vi "数据发送组合-20200825 (子VI).vi"(10 "枚举":T2(ring), 11 "插值后的数组元素":T1) -> (3 "字符串":string)   [LabVIEW 2016, in "数据传输系统.lvlib"]
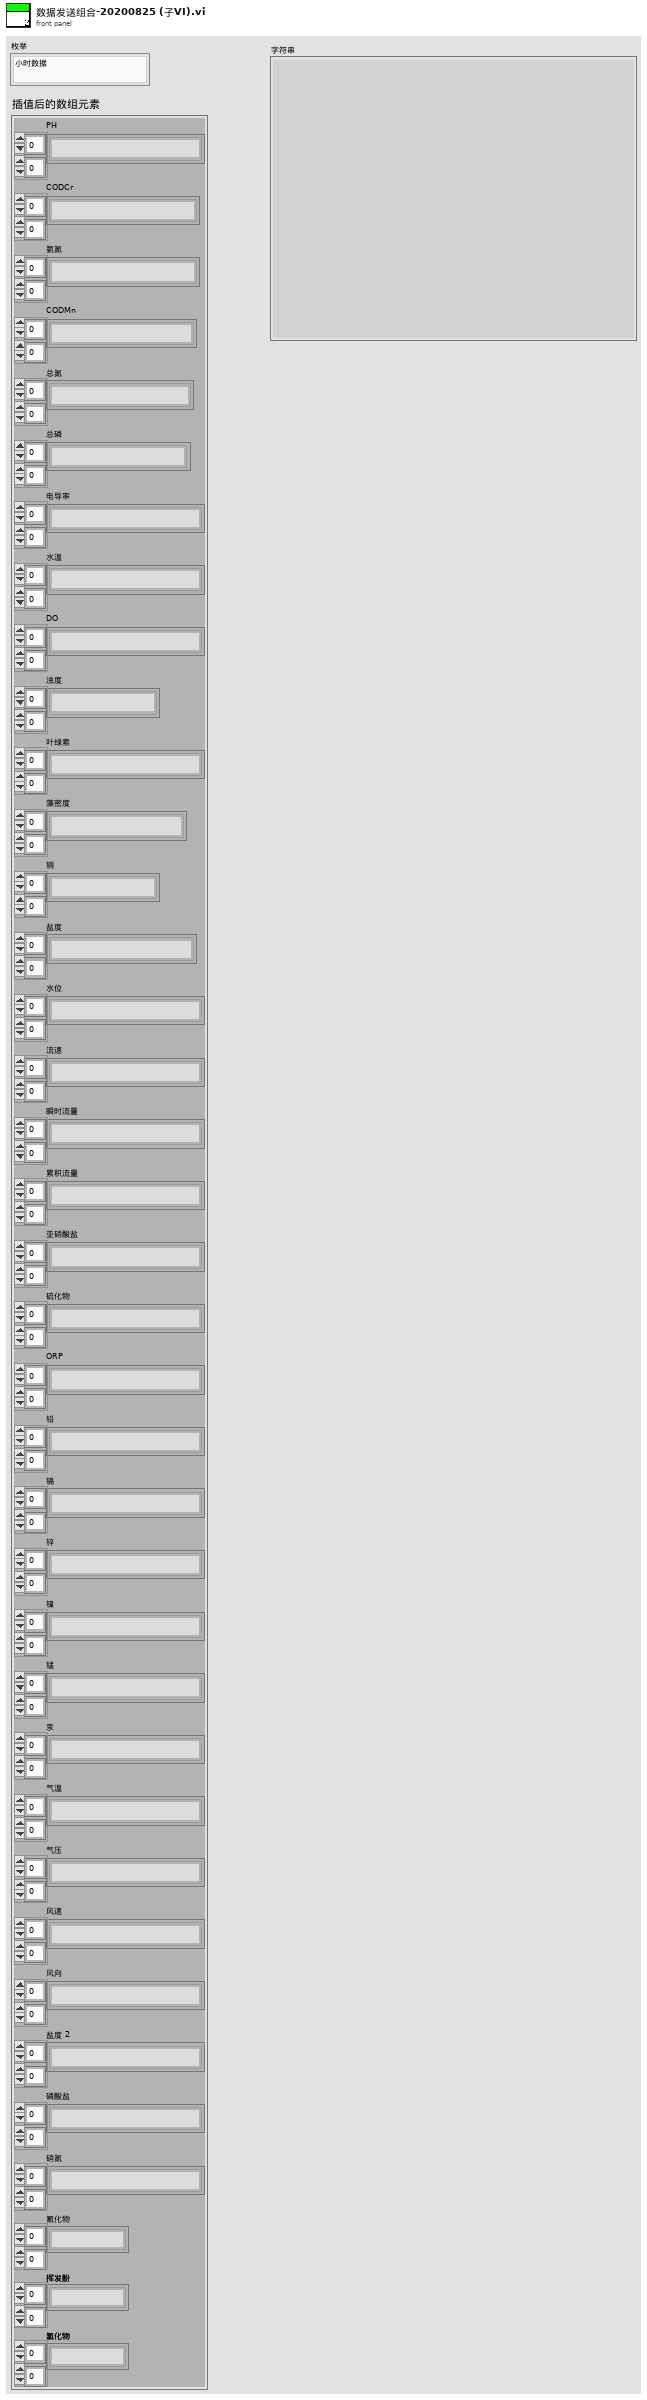
[diagram p1: front panel]
types:
  T1 = cluster{"PH":string[][], "CODCr":string[][], "氨氮":string[][], "CODMn":string[][], "总氮":string[][], "总磷":string[][], "电导率":string[][], "水温":string[][], "DO":string[][], "浊度":string[][], "叶绿素":string[][], "藻密度":string[][], "铜":string[][], "盐度":string[][], "水位":string[][], "流速":string[][], "瞬时流量":string[][], "累积流量":string[][], "亚硝酸盐":string[][], "硫化物":string[][], "ORP":string[][], "铅":string[][], "镉":string[][], "锌":string[][], "镍":string[][], "锰":string[][], "汞":string[][], "气温":string[][], "气压":string[][], "风速":string[][], "风向":string[][], "盐度 2":string[][], "磷酸盐":string[][], "硝氮":string[][], "氟化物":string[][], "挥发酚":string[][], "氯化物":string[][]}
  T2 = enum16{"小时数据", "实时数据", "平行样测试", "集成干预测试", "加标回收测试", "核查数据", "空白零点跨度数据", "提取小时数据", "提取实时数据", "操作日志", "仪器参数", "3090仪器参数", "提取仪器参数", "报警信息"}
  T3 = cluster{"CODMn":dbl, "CODCr":dbl, "DO":dbl, "铜":dbl, "PH":dbl, "氨氮":dbl, "比电导率":dbl, "水温":dbl, "COD":dbl, "浊度":dbl, "总氮":dbl, "总磷":dbl, "叶绿素a":dbl, "藻密度":dbl, "水位":dbl, "流速":dbl, "瞬时流量":dbl, "累积流量":dbl, "亚硝酸盐":dbl, "硫化物":dbl, "ORP":dbl, "铅":dbl, "镉":dbl, "锌":dbl, "镍":dbl, "锰":dbl, "汞":dbl, "气温":dbl, "气压":dbl, "风速":dbl, "风向":dbl, "盐度":dbl, "磷酸盐":dbl, "硝氮":dbl, "氟化物":dbl, "挥发酚":dbl, "氯化物":dbl}
  T4 = cluster{"CODMn":string, "CODCr":string, "DO":string, "铜":string, "PH":string, "氨氮":string, "比电导率":string, "水温":string, "COD":string, "浊度":string, "总氮":string, "总磷":string, "叶绿素a":string, "藻密度":string, "水位":string, "流速":string, "瞬时流量":string, "累积流量":string, "亚硝酸盐":string, "硫化物":string, "ORP":string, "铅":string, "镉":string, "锌":string, "镍":string, "锰":string, "汞":string, "气温":string, "气压":string, "风速":string, "风向":string, "盐度":string, "磷酸盐":string, "硝氮":string, "氟化物":string, "挥发酚":string, "氯化物":string}
  T5 = typedef "数据传输系统.lvlib/应用环境.ctl" = enum16{"STD", "GB212", "婉仪平台"}
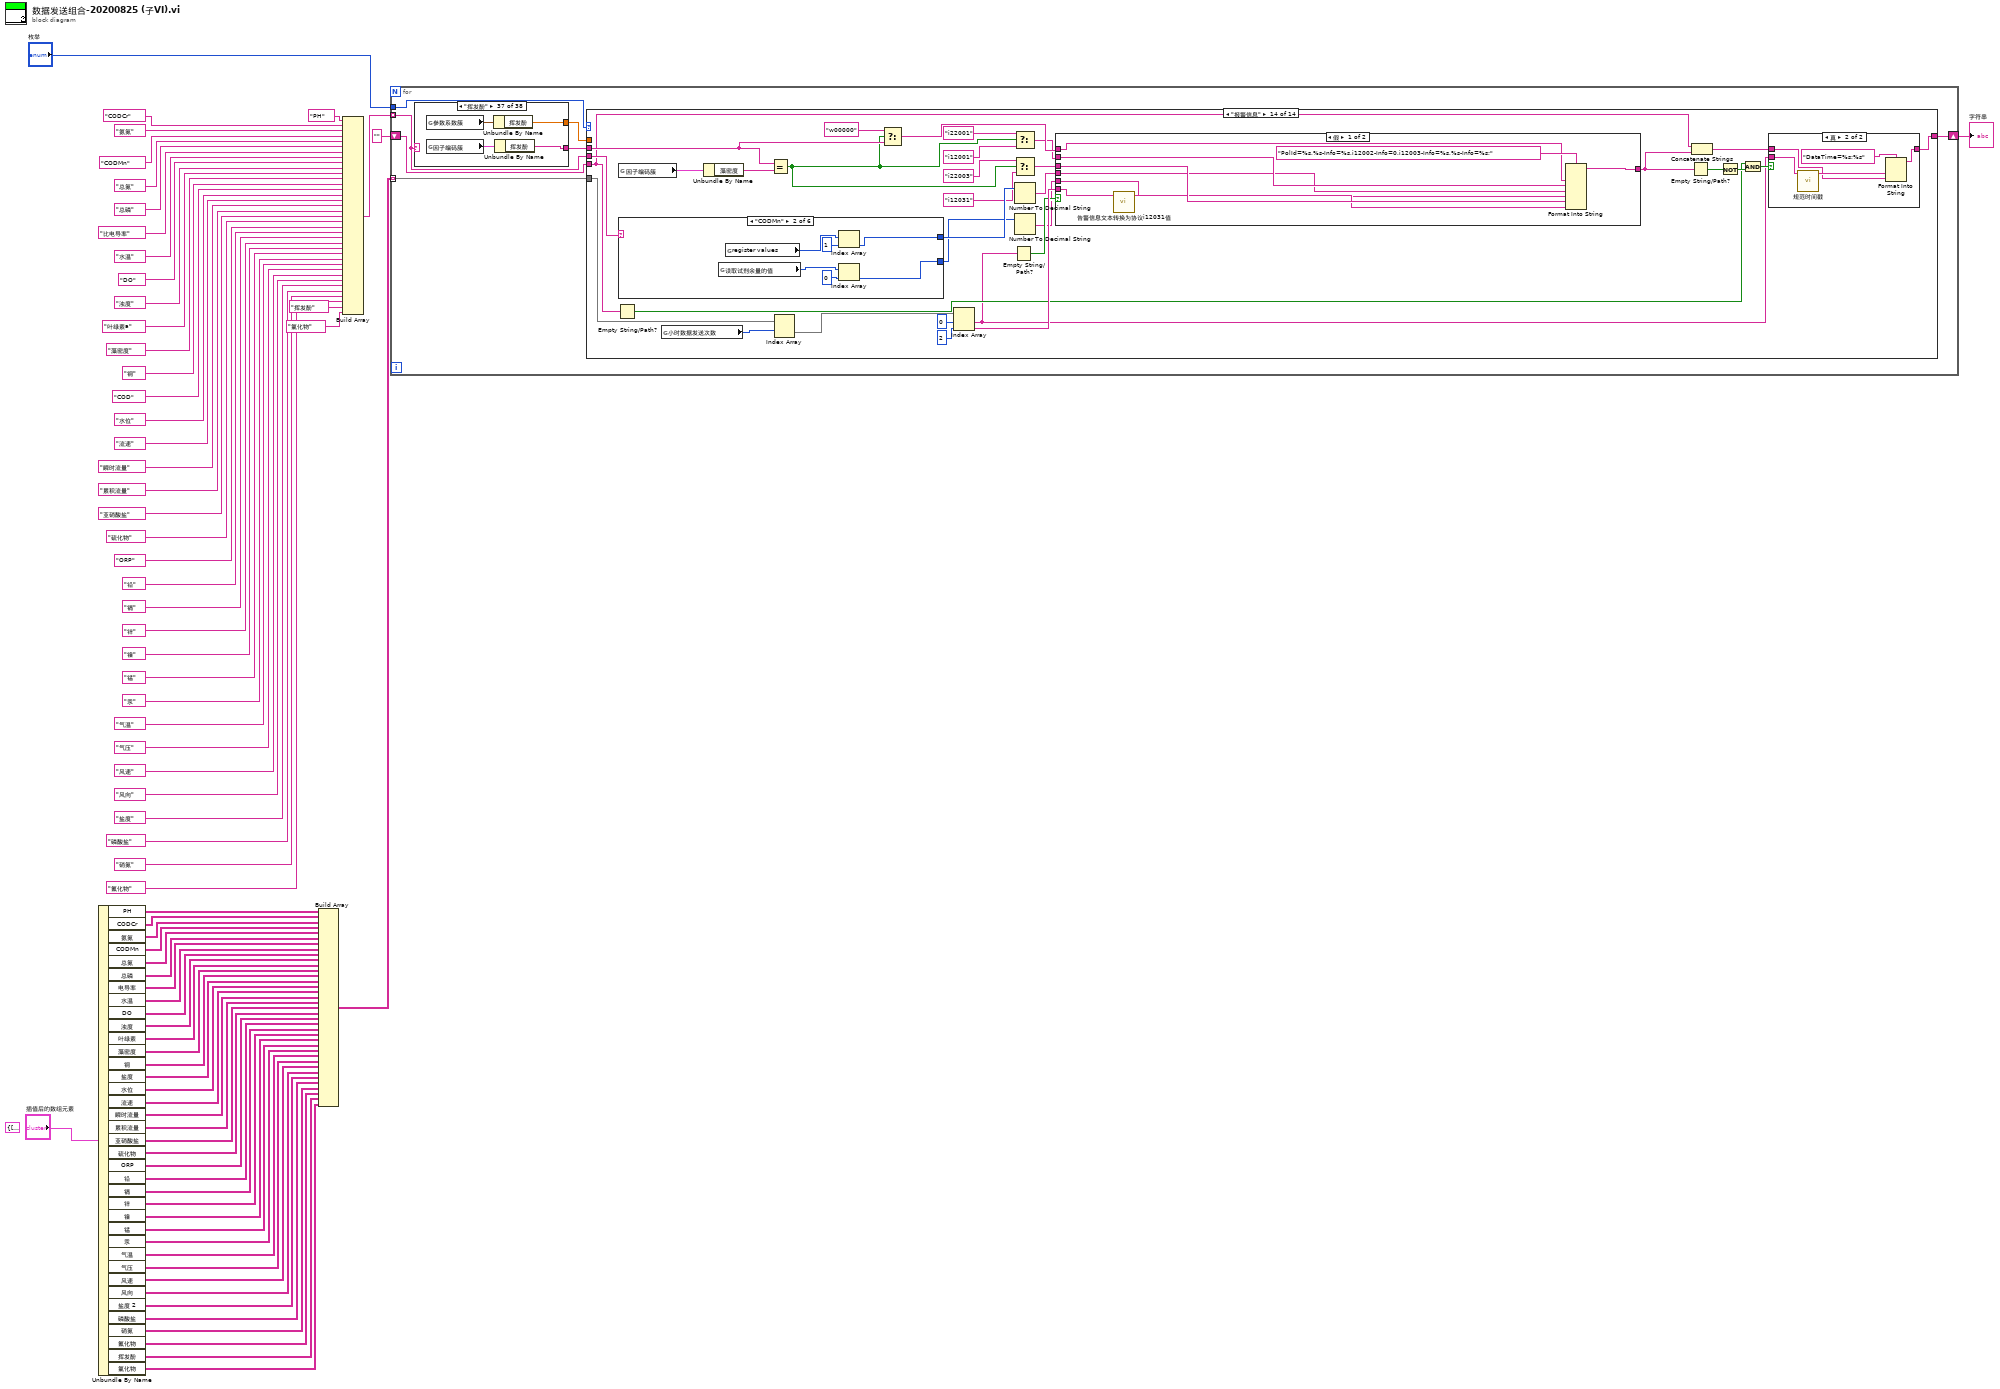
[diagram p0: block diagram]
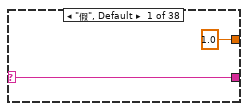
[diagram p2: hidden frame]
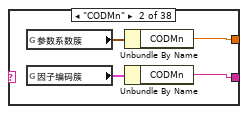
[diagram p3: hidden frame]
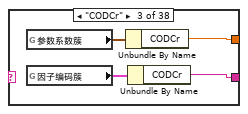
[diagram p4: hidden frame]
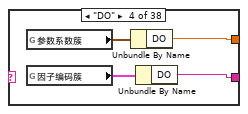
[diagram p5: hidden frame]
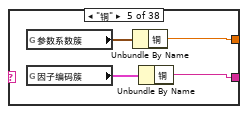
[diagram p6: hidden frame]
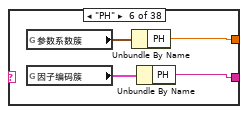
[diagram p7: hidden frame]
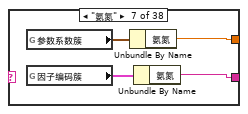
[diagram p8: hidden frame]
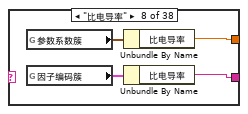
[diagram p9: hidden frame]
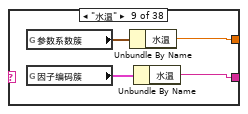
[diagram p10: hidden frame]
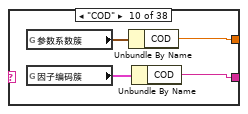
[diagram p11: hidden frame]
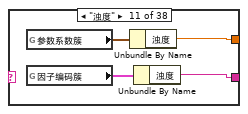
[diagram p12: hidden frame]
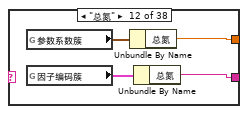
[diagram p13: hidden frame]
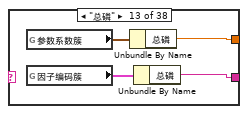
[diagram p14: hidden frame]
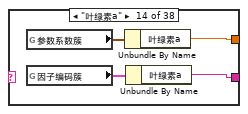
[diagram p15: hidden frame]
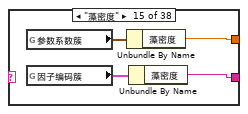
[diagram p16: hidden frame]
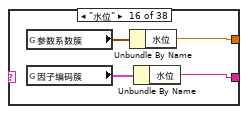
[diagram p17: hidden frame]
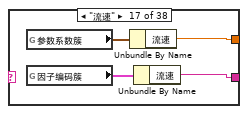
[diagram p18: hidden frame]
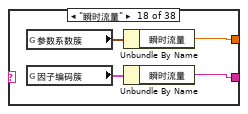
[diagram p19: hidden frame]
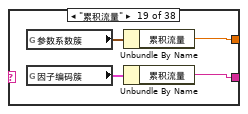
[diagram p20: hidden frame]
diagram:
  (unwired) T1 {"PH"=[], "CODCr"=[], "氨氮"=[], "CODMn"=[], "总氮"=[], "总磷"=[], "电导率"=[], "水温"=[], "DO"=[], "浊度"=[], "叶绿素"=[], "藻密度"=[], "铜"=[], "盐度"=[], "水位"=[], "流速"=[], "瞬时流量"=[], "累积流量"=[], "亚硝酸盐"=[], "硫化物"=[], "ORP"=[], "铅"=[], "镉"=[], "锌"=[], "镍"=[], "锰"=[], "汞"=[], "气温"=[], "气压"=[], "风速"=[], "风向"=[], "盐度 2"=[], "磷酸盐"=[], "硝氮"=[], "氟化物"=[], "挥发酚"=[], "氯化物"=[]} ("插值后的数组元素")
  n1 = Unbundle By Name("插值后的数组元素") -> ("PH"=w80:string[][], "CODCr"=w79:string[][], "氨氮"=w78:string[][], "CODMn"=w77:string[][], "总氮"=w76:string[][], "总磷"=w75:string[][], "电导率"=w74:string[][], "水温"=w73:string[][], "DO"=w72:string[][], "浊度"=w71:string[][], "叶绿素"=w70:string[][], "藻密度"=w69:string[][], "铜"=w68:string[][], "盐度"=w67:string[][], "水位"=w66:string[][], "流速"=w65:string[][], "瞬时流量"=w64:string[][], "累积流量"=w63:string[][], "亚硝酸盐"=w62:string[][], "硫化物"=w61:string[][], "ORP"=w60:string[][], "铅"=w59:string[][], "镉"=w58:string[][], "锌"=w57:string[][], "镍"=w56:string[][], "锰"=w55:string[][], "汞"=w54:string[][], "气温"=w18:string[][], "气压"=w19:string[][], "风速"=w20:string[][], "风向"=w21:string[][], "盐度 2"=w12:string[][], "磷酸盐"=w11:string[][], "硝氮"=w10:string[][], "氟化物"=w6:string[][], "挥发酚"=w4:string[][], "氯化物"=w3:string[][])
  n2 = Build Array(w80, w79, w78, w77, w76, w75, w74, w73, w72, w71, w70, w69, w68, w67, w66, w65, w64, w63, w62, w61, w60, w59, w58, w57, w56, w55, w54, w18, w19, w20, w21, w12, w11, w10, w6, w4, w3) -> (w53:string[][][])
  n3 = Build Array("PH" ("污染物编码"), "CODCr" ("污染物编码"), "氨氮" ("污染物编码"), "CODMn" ("污染物编码"), "总氮" ("污染物编码"), "总磷" ("污染物编码"), "比电导率" ("污染物编码"), "水温" ("污染物编码"), "DO" ("污染物编码"), "浊度" ("污染物编码"), "叶绿素a" ("污染物编码"), "藻密度" ("污染物编码"), "铜" ("污染物编码"), "COD" ("污染物编码"), "水位" ("污染物编码"), "流速" ("污染物编码"), "瞬时流量" ("污染物编码"), "累积流量" ("污染物编码"), "亚硝酸盐" ("污染物编码"), "硫化物" ("污染物编码"), "ORP" ("污染物编码"), "铅" ("污染物编码"), "镉" ("污染物编码"), "锌" ("污染物编码"), "镍" ("污染物编码"), "锰" ("污染物编码"), "汞" ("污染物编码"), "气温" ("污染物编码"), "气压" ("污染物编码"), "风速" ("污染物编码"), "风向" ("污染物编码"), "盐度" ("污染物编码"), "磷酸盐" ("污染物编码"), "硝氮" ("污染物编码"), "氟化物" ("污染物编码"), "挥发酚" ("污染物编码"), "氯化物" ("污染物编码")) -> (w25:string[])
  n4 = for {
    tunnel: w53 -> [w87] mode=indexing
    tunnel: w25 -> [w82] mode=indexing
    shift-right: [w86] -> w23
    shift-left: "" -> [w85]
    tunnel: "枚举" -> [w84]
    n5 = case shown="\"挥发酚\"" w82 {
      selector: w82 -> [w89 _ _ _ _ _ _ _ _ _ _ _ _ _ _ _ _ _ _ _ _ _ _ _ _ _ _ _ _ _ _ _ _ _ _ _ _ _]
      tunnel: [w89 w92 w96 w100 w104 w108 w112 w116 w120 w124 w128 w132 w136 w140 w144 w148 w152 w156 w160 w164 w168 w172 w176 w180 w184 w188 w192 w196 w200 w204 w208 w212 w216 w220 w224 w228 w232 w236] -> w83
      tunnel: [1.0 ("风向") w90 w94 w98 w102 w106 w110 w114 w118 w122 w126 w130 w134 w138 w142 w146 w150 w154 w158 w162 w166 w170 w174 w178 w182 w186 w190 w194 w198 w202 w206 w210 w214 w218 w222 w226 w230 w234] -> w81
      frame "假", Default {
      }
      frame "CODMn" {
        n6 = global read "断电保存全局.vi" "参数系数簇"() -> (w91:T3)
        n7 = global read "断电保存全局.vi" "因子编码簇"() -> (w93:T4)
        n8 = Unbundle By Name(w91) -> ("CODMn"=w90:dbl)
        n9 = Unbundle By Name(w93) -> ("CODMn"=w92:string)
      }
      frame "CODCr" {
        n10 = global read "断电保存全局.vi" "参数系数簇"() -> (w95:T3)
        n11 = global read "断电保存全局.vi" "因子编码簇"() -> (w97:T4)
        n12 = Unbundle By Name(w95) -> ("CODCr"=w94:dbl)
        n13 = Unbundle By Name(w97) -> ("CODCr"=w96:string)
      }
      frame "DO" {
        n14 = global read "断电保存全局.vi" "参数系数簇"() -> (w99:T3)
        n15 = global read "断电保存全局.vi" "因子编码簇"() -> (w101:T4)
        n16 = Unbundle By Name(w99) -> ("DO"=w98:dbl)
        n17 = Unbundle By Name(w101) -> ("DO"=w100:string)
      }
      frame "铜" {
        n18 = global read "断电保存全局.vi" "参数系数簇"() -> (w103:T3)
        n19 = global read "断电保存全局.vi" "因子编码簇"() -> (w105:T4)
        n20 = Unbundle By Name(w103) -> ("铜"=w102:dbl)
        n21 = Unbundle By Name(w105) -> ("铜"=w104:string)
      }
      frame "PH" {
        n22 = global read "断电保存全局.vi" "参数系数簇"() -> (w107:T3)
        n23 = global read "断电保存全局.vi" "因子编码簇"() -> (w109:T4)
        n24 = Unbundle By Name(w107) -> ("PH"=w106:dbl)
        n25 = Unbundle By Name(w109) -> ("PH"=w108:string)
      }
      frame "氨氮" {
        n26 = global read "断电保存全局.vi" "参数系数簇"() -> (w111:T3)
        n27 = global read "断电保存全局.vi" "因子编码簇"() -> (w113:T4)
        n28 = Unbundle By Name(w111) -> ("氨氮"=w110:dbl)
        n29 = Unbundle By Name(w113) -> ("氨氮"=w112:string)
      }
      frame "比电导率" {
        n30 = global read "断电保存全局.vi" "参数系数簇"() -> (w115:T3)
        n31 = global read "断电保存全局.vi" "因子编码簇"() -> (w117:T4)
        n32 = Unbundle By Name(w115) -> ("比电导率"=w114:dbl)
        n33 = Unbundle By Name(w117) -> ("比电导率"=w116:string)
      }
      frame "水温" {
        n34 = global read "断电保存全局.vi" "参数系数簇"() -> (w119:T3)
        n35 = global read "断电保存全局.vi" "因子编码簇"() -> (w121:T4)
        n36 = Unbundle By Name(w119) -> ("水温"=w118:dbl)
        n37 = Unbundle By Name(w121) -> ("水温"=w120:string)
      }
      frame "COD" {
        n38 = global read "断电保存全局.vi" "参数系数簇"() -> (w123:T3)
        n39 = global read "断电保存全局.vi" "因子编码簇"() -> (w125:T4)
        n40 = Unbundle By Name(w123) -> ("COD"=w122:dbl)
        n41 = Unbundle By Name(w125) -> ("COD"=w124:string)
      }
      frame "浊度" {
        n42 = global read "断电保存全局.vi" "参数系数簇"() -> (w127:T3)
        n43 = global read "断电保存全局.vi" "因子编码簇"() -> (w129:T4)
        n44 = Unbundle By Name(w127) -> ("浊度"=w126:dbl)
        n45 = Unbundle By Name(w129) -> ("浊度"=w128:string)
      }
      frame "总氮" {
        n46 = global read "断电保存全局.vi" "参数系数簇"() -> (w131:T3)
        n47 = global read "断电保存全局.vi" "因子编码簇"() -> (w133:T4)
        n48 = Unbundle By Name(w131) -> ("总氮"=w130:dbl)
        n49 = Unbundle By Name(w133) -> ("总氮"=w132:string)
      }
      frame "总磷" {
        n50 = global read "断电保存全局.vi" "参数系数簇"() -> (w135:T3)
        n51 = global read "断电保存全局.vi" "因子编码簇"() -> (w137:T4)
        n52 = Unbundle By Name(w135) -> ("总磷"=w134:dbl)
        n53 = Unbundle By Name(w137) -> ("总磷"=w136:string)
      }
      frame "叶绿素a" {
        n54 = global read "断电保存全局.vi" "参数系数簇"() -> (w139:T3)
        n55 = global read "断电保存全局.vi" "因子编码簇"() -> (w141:T4)
        n56 = Unbundle By Name(w139) -> ("叶绿素a"=w138:dbl)
        n57 = Unbundle By Name(w141) -> ("叶绿素a"=w140:string)
      }
      frame "藻密度" {
        n58 = global read "断电保存全局.vi" "参数系数簇"() -> (w143:T3)
        n59 = global read "断电保存全局.vi" "因子编码簇"() -> (w145:T4)
        n60 = Unbundle By Name(w143) -> ("藻密度"=w142:dbl)
        n61 = Unbundle By Name(w145) -> ("藻密度"=w144:string)
      }
      frame "水位" {
        n62 = global read "断电保存全局.vi" "参数系数簇"() -> (w147:T3)
        n63 = global read "断电保存全局.vi" "因子编码簇"() -> (w149:T4)
        n64 = Unbundle By Name(w147) -> ("水位"=w146:dbl)
        n65 = Unbundle By Name(w149) -> ("水位"=w148:string)
      }
      frame "流速" {
        n66 = global read "断电保存全局.vi" "参数系数簇"() -> (w151:T3)
        n67 = global read "断电保存全局.vi" "因子编码簇"() -> (w153:T4)
        n68 = Unbundle By Name(w151) -> ("流速"=w150:dbl)
        n69 = Unbundle By Name(w153) -> ("流速"=w152:string)
      }
      frame "瞬时流量" {
        n70 = global read "断电保存全局.vi" "参数系数簇"() -> (w155:T3)
        n71 = global read "断电保存全局.vi" "因子编码簇"() -> (w157:T4)
        n72 = Unbundle By Name(w155) -> ("瞬时流量"=w154:dbl)
        n73 = Unbundle By Name(w157) -> ("瞬时流量"=w156:string)
      }
      frame "累积流量" {
        n74 = global read "断电保存全局.vi" "参数系数簇"() -> (w159:T3)
        n75 = global read "断电保存全局.vi" "因子编码簇"() -> (w161:T4)
        n76 = Unbundle By Name(w159) -> ("累积流量"=w158:dbl)
        n77 = Unbundle By Name(w161) -> ("累积流量"=w160:string)
      }
      frame "亚硝酸盐" {
        n78 = global read "断电保存全局.vi" "参数系数簇"() -> (w163:T3)
        n79 = global read "断电保存全局.vi" "因子编码簇"() -> (w165:T4)
        n80 = Unbundle By Name(w163) -> ("亚硝酸盐"=w162:dbl)
        n81 = Unbundle By Name(w165) -> ("亚硝酸盐"=w164:string)
      }
      frame "硫化物" {
        n82 = global read "断电保存全局.vi" "参数系数簇"() -> (w167:T3)
        n83 = global read "断电保存全局.vi" "因子编码簇"() -> (w169:T4)
        n84 = Unbundle By Name(w167) -> ("硫化物"=w166:dbl)
        n85 = Unbundle By Name(w169) -> ("硫化物"=w168:string)
      }
      frame "ORP" {
        n86 = global read "断电保存全局.vi" "参数系数簇"() -> (w171:T3)
        n87 = global read "断电保存全局.vi" "因子编码簇"() -> (w173:T4)
        n88 = Unbundle By Name(w171) -> ("ORP"=w170:dbl)
        n89 = Unbundle By Name(w173) -> ("ORP"=w172:string)
      }
      frame "铅" {
        n90 = global read "断电保存全局.vi" "参数系数簇"() -> (w175:T3)
        n91 = global read "断电保存全局.vi" "因子编码簇"() -> (w177:T4)
        n92 = Unbundle By Name(w175) -> ("铅"=w174:dbl)
        n93 = Unbundle By Name(w177) -> ("铅"=w176:string)
      }
      frame "镉" {
        n94 = global read "断电保存全局.vi" "参数系数簇"() -> (w179:T3)
        n95 = global read "断电保存全局.vi" "因子编码簇"() -> (w181:T4)
        n96 = Unbundle By Name(w179) -> ("镉"=w178:dbl)
        n97 = Unbundle By Name(w181) -> ("镉"=w180:string)
      }
      frame "锌" {
        n98 = global read "断电保存全局.vi" "参数系数簇"() -> (w183:T3)
        n99 = global read "断电保存全局.vi" "因子编码簇"() -> (w185:T4)
        n100 = Unbundle By Name(w183) -> ("锌"=w182:dbl)
        n101 = Unbundle By Name(w185) -> ("锌"=w184:string)
      }
      frame "镍" {
        n102 = global read "断电保存全局.vi" "参数系数簇"() -> (w187:T3)
        n103 = global read "断电保存全局.vi" "因子编码簇"() -> (w189:T4)
        n104 = Unbundle By Name(w187) -> ("镍"=w186:dbl)
        n105 = Unbundle By Name(w189) -> ("镍"=w188:string)
      }
      frame "锰" {
        n106 = global read "断电保存全局.vi" "参数系数簇"() -> (w191:T3)
        n107 = global read "断电保存全局.vi" "因子编码簇"() -> (w193:T4)
        n108 = Unbundle By Name(w191) -> ("锰"=w190:dbl)
        n109 = Unbundle By Name(w193) -> ("锰"=w192:string)
      }
      frame "汞" {
        n110 = global read "断电保存全局.vi" "参数系数簇"() -> (w195:T3)
        n111 = global read "断电保存全局.vi" "因子编码簇"() -> (w197:T4)
        n112 = Unbundle By Name(w195) -> ("汞"=w194:dbl)
        n113 = Unbundle By Name(w197) -> ("汞"=w196:string)
      }
      frame "气温" {
        n114 = global read "断电保存全局.vi" "参数系数簇"() -> (w199:T3)
        n115 = global read "断电保存全局.vi" "因子编码簇"() -> (w201:T4)
        n116 = Unbundle By Name(w199) -> ("气温"=w198:dbl)
        n117 = Unbundle By Name(w201) -> ("气温"=w200:string)
      }
      frame "气压" {
        n118 = global read "断电保存全局.vi" "参数系数簇"() -> (w203:T3)
        n119 = global read "断电保存全局.vi" "因子编码簇"() -> (w205:T4)
        n120 = Unbundle By Name(w203) -> ("气压"=w202:dbl)
        n121 = Unbundle By Name(w205) -> ("气压"=w204:string)
      }
      frame "风速" {
        n122 = global read "断电保存全局.vi" "参数系数簇"() -> (w207:T3)
        n123 = global read "断电保存全局.vi" "因子编码簇"() -> (w209:T4)
        n124 = Unbundle By Name(w207) -> ("风速"=w206:dbl)
        n125 = Unbundle By Name(w209) -> ("风速"=w208:string)
      }
      frame "风向" {
        n126 = global read "断电保存全局.vi" "参数系数簇"() -> (w211:T3)
        n127 = global read "断电保存全局.vi" "因子编码簇"() -> (w213:T4)
        n128 = Unbundle By Name(w211) -> ("风向"=w210:dbl)
        n129 = Unbundle By Name(w213) -> ("风向"=w212:string)
      }
      frame "盐度" {
        n130 = global read "断电保存全局.vi" "参数系数簇"() -> (w215:T3)
        n131 = global read "断电保存全局.vi" "因子编码簇"() -> (w217:T4)
        n132 = Unbundle By Name(w215) -> ("盐度"=w214:dbl)
        n133 = Unbundle By Name(w217) -> ("盐度"=w216:string)
      }
      frame "磷酸盐" {
        n134 = global read "断电保存全局.vi" "参数系数簇"() -> (w219:T3)
        n135 = global read "断电保存全局.vi" "因子编码簇"() -> (w221:T4)
        n136 = Unbundle By Name(w219) -> ("磷酸盐"=w218:dbl)
        n137 = Unbundle By Name(w221) -> ("磷酸盐"=w220:string)
      }
      frame "硝氮" {
        n138 = global read "断电保存全局.vi" "参数系数簇"() -> (w223:T3)
        n139 = global read "断电保存全局.vi" "因子编码簇"() -> (w225:T4)
        n140 = Unbundle By Name(w223) -> ("硝氮"=w222:dbl)
        n141 = Unbundle By Name(w225) -> ("硝氮"=w224:string)
      }
      frame "氟化物" {
        n142 = global read "断电保存全局.vi" "参数系数簇"() -> (w227:T3)
        n143 = global read "断电保存全局.vi" "因子编码簇"() -> (w229:T4)
        n144 = Unbundle By Name(w227) -> ("氟化物"=w226:dbl)
        n145 = Unbundle By Name(w229) -> ("氟化物"=w228:string)
      }
      frame "挥发酚" {
        n146 = global read "断电保存全局.vi" "参数系数簇"() -> (w231:T3)
        n147 = global read "断电保存全局.vi" "因子编码簇"() -> (w233:T4)
        n148 = Unbundle By Name(w231) -> ("挥发酚"=w230:dbl)
        n149 = Unbundle By Name(w233) -> ("挥发酚"=w232:string)
      }
      frame "氯化物" {
        n150 = global read "断电保存全局.vi" "参数系数簇"() -> (w235:T3)
        n151 = global read "断电保存全局.vi" "因子编码簇"() -> (w237:T4)
        n152 = Unbundle By Name(w235) -> ("氯化物"=w234:dbl)
        n153 = Unbundle By Name(w237) -> ("氯化物"=w236:string)
      }
    }
    n154 = case shown="\"报警信息\"" w84 {
      tunnel: w87 -> [w252 w297 w328 w337 w392 w398 w410 w434 w456 w493 w511 w518 w528 w550]
      tunnel: w83 -> [w248 w290 w327 w338 w388 w397 w409 w428 w455 w481 w509 w516 w527 w553]
      tunnel: [w251 w294 w329 w335 w393 w394 w406 w425 w454 w488 w506 w515 w523 w539] -> w86
      tunnel: w85 -> [w250 w295 w331 w336 w389 w396 w407 w426 w457 w489 w507 w517 w524 w534]
      tunnel: w82 -> [w246 w289 _ w332 _ _ _ _ _ _ _ _ _ w548]
      tunnel: w81 -> [w243 w285 _ w333 _ _ _ w421 w450 _ _ _ _ _]
      frame "小时数据", Default {
        n155 = global read "全局 小时数据发送次数.vi" "小时数据发送次数"() -> (w255:i32)
        n156 = Index Array(array=w252, index (row)=w255) -> (element=w254:string[])  [unwired: 1 in]
        n157 = case shown="\"\", 默认" w246 {
          tunnel: w254 -> [w267 w270]
          tunnel: [w264 w268] -> w244
          tunnel: ["N" ("字符串") w269] -> w240
          frame "风速", "风向", "累积流量", "流速", "气温", "气压", "水位", "瞬时流量" {
            n158 = Index Array(array=w267, index=1 ("索引")) -> (element=w264:string)
          }
          frame "", Default {
            n159 = Index Array(array=w270, index #1=2 ("索引"), index #2=3 ("索引"), index #3=5 ("索引")) -> (element #1=w273:string, element #2=w272:string, element #3=w269:string)
            n160 = case shown="\"N\", 默认" w273 {
              tunnel: [w276 ""] -> w268
              tunnel: w272 -> [w276 _]
              frame "N", Default {
              }
              frame "M" {
              }
            }
          }
        }
        n161 = Empty String/Path?(string/path=w244) -> (empty?=w245:bool)
        n162 = case shown="假" w245 {
          tunnel: w244 -> [w261 w263]
          tunnel: w243 -> [w260 _]
          tunnel: [w258 w263] -> w242
          frame False {
            n163 = Fract/Exp String To Number(string=w261) -> (number=w262:dbl)  [unwired: 3 in, 1 out]
            n164 = Multiply(x=w262, y=w260) -> (x*y=w259:dbl)
            n165 = Number To Fractional String(number=w259) -> (F-format string=w258:string)  [unwired: 3 in]
          }
          frame True {
            # "空"
          }
        }
        n166 = global read "断电保存全局.vi" "地表水/污染源"() -> (w241:bool)
        n167 = call "数据编码整合输出.vi"("数据标识"=w240, "数据类型"="-Avg=", "污染物编码"=w248, "地表水/污染源"=w241, "数据值"=w242) -> ("编码输出"=w239:string)  [unwired: 6 in]
        n168 = case shown="\"pf\"" w240 {
          tunnel: w239 -> [w256 _]
          tunnel: [w256 ""] -> w238
          frame "假", Default {
          }
          frame "pf" {
            # "pf不传小时数据"
          }
        }
        n169 = global read "断电保存全局.vi" "数据发送协议"() -> (w249:enum16{"2005-212协议", "2017-212协议"})
        n170 = case shown="\"2017-212协议\"" w249 {
          tunnel: w246 -> [w280 _]
          tunnel: w238 -> [w278 w283]
          tunnel: [w279 w283] -> w247
          frame "2005-212协议", Default {
            n171 = case shown="\"风速\", \"风向\", \"累积流量\", \"流速\", \"气温\", \"气压\", \"水位\"" w280 {
              tunnel: [w281 ""] -> w279
              tunnel: w278 -> [w281 _]
              frame "假", Default {
              }
              frame "风速", "风向", "累积流量", "流速", "气温", "气压", "水位" {
              }
            }
          }
          frame "2017-212协议" {
          }
        }
        n172 = Concatenate Strings(w250, w247) -> (w251:string)
      }
      frame "实时数据" {
        n173 = global read "全局 小时数据发送次数.vi" "小时数据发送次数"() -> (w298:i32)
        n174 = Index Array(array=w297, index (row)=w298) -> (element=w299:string[])  [unwired: 1 in]
        n175 = case shown="\"\", 默认" w289 {
          tunnel: w299 -> [w308 w312 w318]
          tunnel: [w307 w311 w317] -> w287
          tunnel: ["N" ("字符串") "N" ("字符串") w315] -> w296
          frame "累积流量", "流速", "水位", "瞬时流量" {
            n176 = Index Array(array=w308, index=1 ("索引")) -> (element=w307:string)
          }
          frame "风速", "风向", "气温", "气压" {
            n177 = Index Array(array=w312, index=1 ("索引")) -> (element=w311:string)
          }
          frame "", Default {
            n178 = Index Array(array=w318, index #1=3 ("索引"), index #2=5 ("索引")) -> (element #1=w317:string, element #2=w315:string)
          }
        }
        n179 = Empty String/Path?(string/path=w287) -> (empty?=w288:bool)
        n180 = case shown="假" w288 {
          tunnel: w287 -> [w304 w306]
          tunnel: w285 -> [w303 _]
          tunnel: [w301 w306] -> w286
          frame False {
            n181 = Fract/Exp String To Number(string=w304) -> (number=w305:dbl)  [unwired: 3 in, 1 out]
            n182 = Multiply(x=w305, y=w303) -> (x*y=w302:dbl)
            n183 = Number To Fractional String(number=w302) -> (F-format string=w301:string)  [unwired: 3 in]
          }
          frame True {
            # "空"
          }
        }
        n184 = global read "断电保存全局.vi" "数据发送协议"() -> (w293:enum16{"2005-212协议", "2017-212协议"})
        n185 = call "数据编码整合输出.vi"("数据标识"=w296, "数据类型"="-Rtd=", "污染物编码"=w290, "地表水/污染源"=FALSE, "数据值"=w286) -> ("编码输出"=w292:string)  [unwired: 6 in]
        n186 = case shown="\"2017-212协议\"" w293 {
          tunnel: w289 -> [w322 _]
          tunnel: w292 -> [w320 w325]
          tunnel: [w321 w325] -> w291
          frame "2005-212协议", Default {
            n187 = case shown="\"假\", 默认" w322 {
              tunnel: [w323 ""] -> w321
              tunnel: w320 -> [w323 _]
              frame "假", Default {
              }
              frame "风速", "风向", "累积流量", "流速", "气温", "气压", "水位" {
              }
            }
          }
          frame "2017-212协议" {
          }
        }
        n188 = Concatenate Strings(w295, w291) -> (w294:string)
      }
      frame "平行样测试" {
        n189 = global read "全局 小时数据发送次数.vi" "小时数据发送次数"() -> (w326:i32)
        n190 = call "平行样集成干预数据组合(子VI).vi"("污染物编码"=w327, "数据输入"=w328, "小时数据发送次数"=w326) -> ("输出组合"=w330:string)  [unwired: 8 in]
        n191 = Concatenate Strings(w331, w330) -> (w329:string)
      }
      frame "集成干预测试" {
        n192 = global read "断电保存全局.vi" "应用环境"() -> (w334:T5)
        n193 = case shown="\"GB212\", 默认" w334 {
          tunnel: w338 -> [w342 w348]
          tunnel: w337 -> [w341 w349]
          tunnel: w336 -> [w340 w350]
          tunnel: [w339 w345] -> w335
          tunnel: w333 -> [_ w347]
          tunnel: w332 -> [_ w346]
          frame "STD" {
            n194 = global read "全局 小时数据发送次数.vi" "小时数据发送次数"() -> (w343:i32)
            n195 = call "平行样集成干预数据组合(子VI).vi"("污染物编码"=w342, "数据输入"=w341, "小时数据发送次数"=w343) -> ("输出组合"=w344:string)  [unwired: 8 in]
            n196 = Concatenate Strings(w340, w344) -> (w339:string)
          }
          frame "GB212", Default {
            n197 = global read "全局 小时数据发送次数.vi" "小时数据发送次数"() -> (w361:i32)
            n198 = Index Array(array=w349, index (row)=w361) -> (element=w360:string[])  [unwired: 1 in]
            n199 = case shown="\"\", 默认" w346 {
              tunnel: w360 -> [w371 w374]
              tunnel: [w368 w373] -> w353
              tunnel: ["N" ("字符串") w372] -> w358
              frame "风速", "风向", "累积流量", "流速", "气温", "气压", "水位", "瞬时流量" {
                n200 = Index Array(array=w371, index=1 ("索引")) -> (element=w368:string)
              }
              frame "", Default {
                n201 = Index Array(array=w374, index #1=2 ("索引"), index #2=3 ("索引"), index #3=5 ("索引")) -> (element #1=w377:string, element #2=w376:string, element #3=w372:string)
                n202 = case shown="\"N\", 默认" w377 {
                  tunnel: [w380 ""] -> w373
                  tunnel: w376 -> [w380 _]
                  frame "N", Default {
                  }
                  frame "M" {
                  }
                }
              }
            }
            n203 = Empty String/Path?(string/path=w353) -> (empty?=w354:bool)
            n204 = case shown="假" w354 {
              tunnel: w353 -> [w365 w367]
              tunnel: w347 -> [w364 _]
              tunnel: [w362 w367] -> w352
              frame False {
                n205 = Fract/Exp String To Number(string=w365) -> (number=w366:dbl)  [unwired: 3 in, 1 out]
                n206 = Multiply(x=w366, y=w364) -> (x*y=w363:dbl)
                n207 = Number To Fractional String(number=w363) -> (F-format string=w362:string)  [unwired: 3 in]
              }
              frame True {
                # "空"
              }
            }
            n208 = global read "断电保存全局.vi" "地表水/污染源"() -> (w351:bool)
            n209 = global read "断电保存全局.vi" "数据发送协议"() -> (w357:enum16{"2005-212协议", "2017-212协议"})
            n210 = call "数据编码整合输出.vi"("数据标识"=w358, "数据类型"="-Avg=", "污染物编码"=w348, "地表水/污染源"=w351, "数据值"=w352) -> ("编码输出"=w356:string)  [unwired: 6 in]
            n211 = case shown="\"2017-212协议\"" w357 {
              tunnel: w346 -> [w384 _]
              tunnel: w356 -> [w382 w387]
              tunnel: [w383 w387] -> w355
              frame "2005-212协议", Default {
                n212 = case shown="\"假\", 默认" w384 {
                  tunnel: [w385 ""] -> w383
                  tunnel: w382 -> [w385 _]
                  frame "假", Default {
                  }
                  frame "风速", "风向", "累积流量", "流速", "气温", "气压", "水位" {
                  }
                }
              }
              frame "2017-212协议" {
              }
            }
            n213 = Concatenate Strings(w350, w355) -> (w345:string)
          }
        }
      }
      frame "加标回收测试" {
        n214 = global read "全局 小时数据发送次数.vi" "小时数据发送次数"() -> (w391:i32)
        n215 = call "加标回收数据组合 (子VI).vi"("小时数据发送次数"=w391, "数据"=w392, "污染物编码"=w388) -> ("组合输出"=w390:string)  [unwired: 7 in, 1 out]
        n216 = Concatenate Strings(w389, w390) -> (w393:string)
      }
      frame "核查数据" {
        n217 = global read "全局 小时数据发送次数.vi" "小时数据发送次数"() -> (w399:i32)
        n218 = call "标样核查数据组合(子VI).vi"("小时数据发送次数"=w399, "数据输入"=w398, "污染物编码"=w397) -> ("输出组合"=w395:string)  [unwired: 8 in]
        n219 = Concatenate Strings(w396, w395) -> (w394:string)
      }
      frame "空白零点跨度数据" {
        n220 = global read "全局 小时数据发送次数.vi" "小时数据发送次数"() -> (w412:i32)
        n221 = Index Array(array=w410, index (row)=w412) -> (element=w416:string[])  [unwired: 1 in]
        n222 = Index Array(array=w416, index #1=0 ("索引"), index #2=3 ("索引"), index #3=6 ("索引"), index #4=7 ("索引"), index #5=5 ("索引")) -> (element #2=w411:string, element #3=w413:string, element #4=w402:string, element #5=w400:string)  [unwired: 1 out]
        n223 = Empty String/Path?(string/path=w402) -> (empty?=w404:bool)
        n224 = case shown="假" w404 {
          tunnel: [w418 "0" ("span value")] -> w403
          tunnel: w402 -> [w418 _]
          frame False {
          }
          frame True {
          }
        }
        n225 = call "零点跨度数据组合 (子VI).vi"("数据标识"=w400, "span value"=w403, "standard value"=w413, "check value"=w411, "污染物编码"=w409) -> ("组合输出"=w408:string)  [unwired: 6 in]
        n226 = Concatenate Strings(w407, w408) -> (w406:string)
      }
      frame "提取小时数据" {
        n227 = global read "全局 小时数据发送次数.vi" "小时数据发送次数"() -> (w435:i32)
        n228 = Index Array(array=w434, index (row)=w435) -> (element=w433:string[])  [unwired: 1 in]
        n229 = Index Array(array=w433, index #2=1 ("索引")) -> (element #2=w422:string)  [unwired: 1 in, 1 out]
        n230 = Empty String/Path?(string/path=w422) -> (empty?=w424:bool)
        n231 = case shown="假" w424 {
          tunnel: w422 -> [w440 w442]
          tunnel: w421 -> [w439 _]
          tunnel: [w437 w442] -> w423
          frame False {
            n232 = Fract/Exp String To Number(string=w440) -> (number=w441:dbl)  [unwired: 3 in, 1 out]
            n233 = Multiply(x=w441, y=w439) -> (x*y=w438:dbl)
            n234 = Number To Fractional String(number=w438) -> (F-format string=w437:string)  [unwired: 3 in]
          }
          frame True {
            # "空"
          }
        }
        n235 = global read "断电保存全局.vi" "地表水/污染源"() -> (w420:bool)
        n236 = global read "断电保存全局.vi" "数据发送协议"() -> (w430:enum16{"2005-212协议", "2017-212协议"})
        n237 = call "数据编码整合输出.vi"("数据标识"="N", "数据类型"="-Avg=", "污染物编码"=w428, "地表水/污染源"=w420, "数据值"=w423) -> ("编码输出"=w427:string)  [unwired: 6 in]
        n238 = case shown="\"2005-212协议\", 默认" w430 {
          tunnel: w428 -> [w445 _]
          tunnel: w427 -> [w443 w448]
          tunnel: [w444 w448] -> w429
          frame "2005-212协议", Default {
            n239 = case shown="\"假\", 默认" w445 {
              tunnel: [w446 ""] -> w444
              tunnel: w443 -> [w446 _]
              frame "假", Default {
              }
              frame "累积流量", "流速", "水位" {
              }
            }
          }
          frame "2017-212协议" {
          }
        }
        n240 = Concatenate Strings(w426, w429) -> (w425:string)
      }
      frame "提取实时数据" {
        n241 = global read "全局 小时数据发送次数.vi" "小时数据发送次数"() -> (w463:i32)
        n242 = Index Array(array=w456, index (row)=w463) -> (element=w464:string[])  [unwired: 1 in]
        n243 = Index Array(array=w464, index #1=3 ("索引"), index #2=5 ("索引")) -> (element #1=w451:string, element #2=w461:string)
        n244 = Empty String/Path?(string/path=w451) -> (empty?=w453:bool)
        n245 = case shown="假" w453 {
          tunnel: w451 -> [w470 w472]
          tunnel: w450 -> [w469 _]
          tunnel: [w467 w472] -> w452
          frame False {
            n246 = Fract/Exp String To Number(string=w470) -> (number=w471:dbl)  [unwired: 3 in, 1 out]
            n247 = Multiply(x=w471, y=w469) -> (x*y=w468:dbl)
            n248 = Number To Fractional String(number=w468) -> (F-format string=w467:string)  [unwired: 3 in]
          }
          frame True {
            # "空"
          }
        }
        n249 = global read "断电保存全局.vi" "地表水/污染源"() -> (w449:bool)
        n250 = global read "断电保存全局.vi" "数据发送协议"() -> (w460:enum16{"2005-212协议", "2017-212协议"})
        n251 = call "数据编码整合输出.vi"("数据标识"=w461, "数据类型"="-Rtd=", "污染物编码"=w455, "地表水/污染源"=w449, "数据值"=w452) -> ("编码输出"=w459:string)  [unwired: 6 in]
        n252 = case shown="\"2017-212协议\"" w460 {
          tunnel: w455 -> [w475 _]
          tunnel: w459 -> [w473 w478]
          tunnel: [w474 w478] -> w458
          frame "2005-212协议", Default {
            n253 = case shown="\"累积流量\", \"流速\", \"水位\"" w475 {
              tunnel: [w476 ""] -> w474
              tunnel: w473 -> [w476 _]
              frame "假", Default {
              }
              frame "累积流量", "流速", "水位" {
              }
            }
          }
          frame "2017-212协议" {
          }
        }
        n254 = Concatenate Strings(w457, w458) -> (w454:string)
      }
      frame "操作日志" {
        n255 = global read "断电保存全局.vi" "因子编码簇"() -> (w484:T4)
        n256 = global read "全局 小时数据发送次数.vi" "小时数据发送次数"() -> (w497:i32)
        n257 = Unbundle By Name(w484) -> ("DO"=w483:string)
        n258 = Equal?(x=w481, y=w483) -> (x = y?=w479:bool)
        n259 = Index Array(array=w493, index (row)=w497) -> (element=w492:string[])  [unwired: 1 in]
        n260 = Index Array(array=w492, index #1=0 ("索引"), index #2=2 ("索引")) -> (element #2=w491:string)  [unwired: 1 out]
        n261 = Empty String/Path?(string/path=w491) -> (empty?=w496:bool)
        n262 = Select(t="w00000", s=w479, f=w481) -> (s? t:f=w480:string)
        n263 = Select(t="i21001", s=w479, f="i11001") -> (s? t:f=w485:string)
        n264 = case shown="假" w496 {
          tunnel: [w501 ""] -> w490
          tunnel: w491 -> [w499 _]
          tunnel: w480 -> [w500 _]
          tunnel: w485 -> [w498 _]
          frame False {
            n265 = Format Into String(format string="PolId=%s,%s-Info=//%s//;" ("格式字符串"), w500, w498, w499) -> (resulting string=w501:string)  [unwired: 2 in, 1 out]
          }
          frame True {
          }
        }
        n266 = Concatenate Strings(w489, w490) -> (w488:string)
      }
      frame "仪器参数" {
        n267 = global read "断电保存全局.vi" "应用环境"() -> (w505:T5)
        n268 = global read "全局 小时数据发送次数.vi" "小时数据发送次数"() -> (w512:i32)
        n269 = case shown="\"GB212\", 默认" w505 {
          tunnel: ["3090仪器参数" ("table") "仪器参数" ("table")] -> w504
          frame "STD" {
          }
          frame "GB212", Default {
          }
        }
        n270 = Index Array(array=w511, index (row)=w512) -> (element=w510:string[])  [unwired: 1 in]
        n271 = call "关键参数组合 (子VI).vi"("table"=w504, "因子编码"=w509, "data"=w510) -> ("字符串"=w508:string)  [unwired: 8 in]
        n272 = Concatenate Strings(w507, w508) -> (w506:string)
      }
      frame "3090仪器参数" {
        n273 = global read "全局 小时数据发送次数.vi" "小时数据发送次数"() -> (w522:i32)
        n274 = Index Array(array=w518, index (row)=w522) -> (element=w520:string[])  [unwired: 1 in]
        n275 = call "关键参数组合 (子VI).vi"("table"="3090仪器参数", "因子编码"=w516, "data"=w520) -> ("字符串"=w519:string)  [unwired: 8 in]
        n276 = Concatenate Strings(w517, w519) -> (w515:string)
      }
      frame "提取仪器参数" {
        n277 = global read "全局 小时数据发送次数.vi" "小时数据发送次数"() -> (w529:i32)
        n278 = Index Array(array=w528, index (row)=w529) -> (element=w526:string[])  [unwired: 1 in]
        n279 = call "提取仪器参数 (子VI).vi"("因子编码"=w527, "数据输入"=w526) -> ("字符串"=w525:string)  [unwired: 9 in]
        n280 = Concatenate Strings(w524, w525) -> (w523:string)
      }
      frame "报警信息" {
        n281 = Empty String/Path?(string/path=w534) -> (empty?=w533:bool)
        n282 = global read "断电保存全局.vi" "因子编码簇"() -> (w556:T4)
        n283 = case shown="\"CODMn\"" w548 {
          tunnel: [u16 0 ("register") w574 w580 w586 w592 w598] -> w546
          tunnel: [u16 0 ("register") w571 w577 w583 w589 w595] -> w531
          frame "假", Default {
          }
          frame "CODMn" {
            n284 = global read "全局1.vi" "读取试剂余量的值"() -> (w572:u16[])
            n285 = global read "全局1.vi" "register values"() -> (w576:u16[])
            n286 = Index Array(array=w576, index=1 ("索引")) -> (element=w574:u16)
            n287 = Index Array(array=w572, index=0 ("索引")) -> (element=w571:u16)
          }
          frame "氨氮" {
            n288 = global read "全局1.vi" "读取试剂余量的值"() -> (w578:u16[])
            n289 = global read "全局1.vi" "register values"() -> (w582:u16[])
            n290 = Index Array(array=w582, index=2 ("索引")) -> (element=w580:u16)
            n291 = Index Array(array=w578, index=1 ("索引")) -> (element=w577:u16)
          }
          frame "总磷" {
            n292 = global read "全局1.vi" "读取试剂余量的值"() -> (w584:u16[])
            n293 = global read "全局1.vi" "register values"() -> (w588:u16[])
            n294 = Index Array(array=w588, index=3 ("索引")) -> (element=w586:u16)
            n295 = Index Array(array=w584, index=2 ("索引")) -> (element=w583:u16)
          }
          frame "总氮" {
            n296 = global read "全局1.vi" "读取试剂余量的值"() -> (w590:u16[])
            n297 = global read "全局1.vi" "register values"() -> (w594:u16[])
            n298 = Index Array(array=w594, index=4 ("索引")) -> (element=w592:u16)
            n299 = Index Array(array=w590, index=3 ("索引")) -> (element=w589:u16)
          }
          frame "CODCr" {
            n300 = global read "全局1.vi" "读取试剂余量的值"() -> (w596:u16[])
            n301 = global read "全局1.vi" "register values"() -> (w600:u16[])
            n302 = Index Array(array=w600, index=5 ("索引")) -> (element=w598:u16)
            n303 = Index Array(array=w596, index=4 ("索引")) -> (element=w595:u16)
          }
        }
        n304 = global read "全局 小时数据发送次数.vi" "小时数据发送次数"() -> (w551:i32)
        n305 = Unbundle By Name(w556) -> ("藻密度"=w555:string)
        n306 = Equal?(x=w553, y=w555) -> (x = y?=w543:bool)
        n307 = Index Array(array=w550, index (row)=w551) -> (element=w549:string[])  [unwired: 1 in]
        n308 = Select(t="w00000", s=w543, f=w553) -> (s? t:f=w552:string)
        n309 = Index Array(array=w549, index #1=0 ("索引"), index #2=2 ("索引")) -> (element #1=w530:string, element #2=w562:string)
        n310 = Empty String/Path?(string/path=w530) -> (empty?=w561:bool)
        n311 = Select(t="i22001", s=w543, f="i12001") -> (s? t:f=w542:string)
        n312 = Select(t="i22003", s=w543, f="i12031") -> (s? t:f=w541:string)
        n313 = Number To Decimal String(number=w546) -> (decimal integer string=w547:string)  [unwired: 1 in]
        n314 = Number To Decimal String(number=w531) -> (decimal integer string=w532:string)  [unwired: 1 in]
        n315 = case shown="假" w561 {
          tunnel: [w609 _] -> w538
          tunnel: w562 -> [w606 _]
          tunnel: w552 -> [w604 _]
          tunnel: w547 -> [w602 _]
          tunnel: w542 -> [w603 _]
          tunnel: w541 -> [w607 _]
          tunnel: w532 -> [w601 _]
          frame False {
            n316 = call "告警信息文本转换为协议i12031值.vi"("字符串"=w606) -> ("十进制整型字符串"=w605:string)  [unwired: 10 in]
            n317 = Format Into String(format string="PolId=%s,%s-Info=%s,i12002-Info=0,i12003-Info=%s,%s-Info=%s;" ("格式字符串"), w604, w603, w602, w601, w607, w605) -> (resulting string=w609:string)  [unwired: 2 in, 1 out]
          }
          frame True {
          }
        }
        n318 = Empty String/Path?(string/path=w538) -> (empty?=w537:bool)
        n319 = Concatenate Strings(w534, w538) -> (w540:string)
        n320 = Not(x=w537) -> (.not. x?=w536:bool)
        n321 = And(x=w533, y=w536) -> (x .and. y?=w535:bool)
        n322 = case shown="真" w535 {
          tunnel: w530 -> [_ w566]
          tunnel: w540 -> [w563 w565]
          tunnel: [w563 w564] -> w539
          frame False {
          }
          frame True {
            n323 = call "规范时间戳.vi"("字符串"=w566) -> ("result string"=w568:string)  [unwired: 10 in]
            n324 = Format Into String(format string="DataTime=%s;%s", w568, w565) -> (resulting string=w564:string)  [unwired: 2 in, 1 out]
          }
        }
      }
    }
  }
  "字符串" <- w23
